vi "Data_folder_Path.vi"(1 "seconds":dbl, 2 "ProjectNumberIn":string, 3 "SetProjectNumber":bool, 4 "FlushHierarchy":bool, 5 "Data Type":string) -> (0 "Data Folder":path)   [LabVIEW 2010]
uses:
  Globals/Constants_global.vi
  Globals/Preference_global.vi
panel:
  out "ProjectNo":string
  out "Hierarchy":string[](array[string])
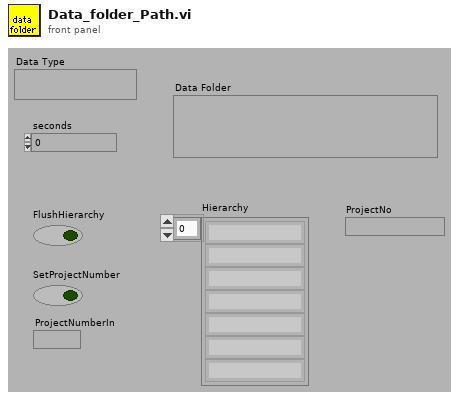
[diagram p1: front panel]
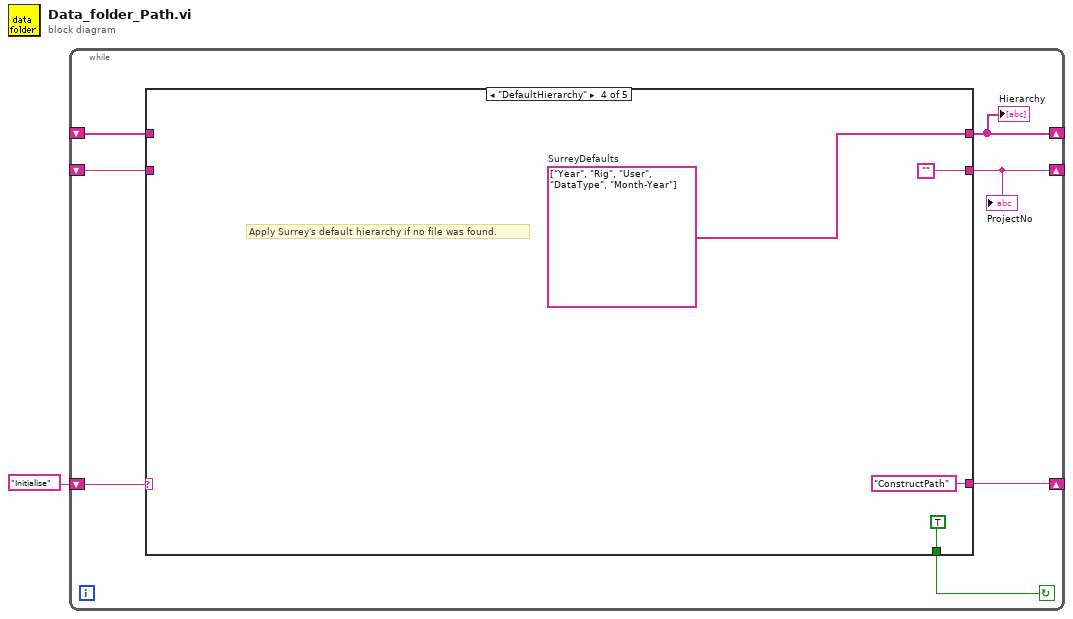
[diagram p0: block diagram]
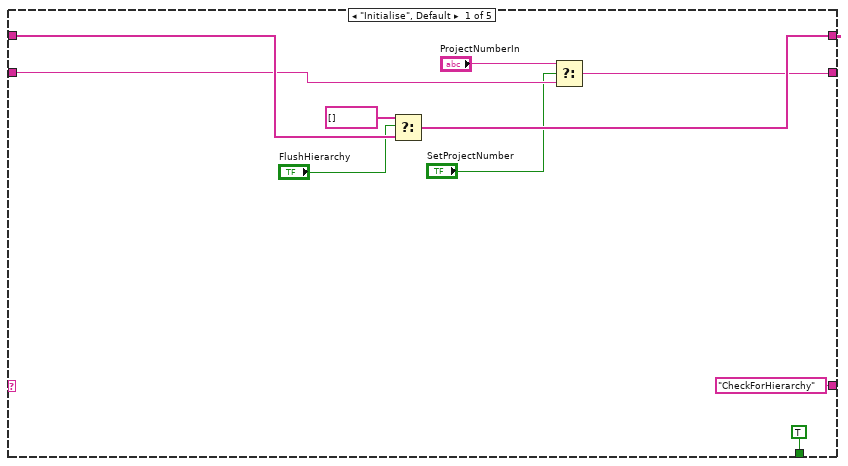
[diagram p2: hidden frame]
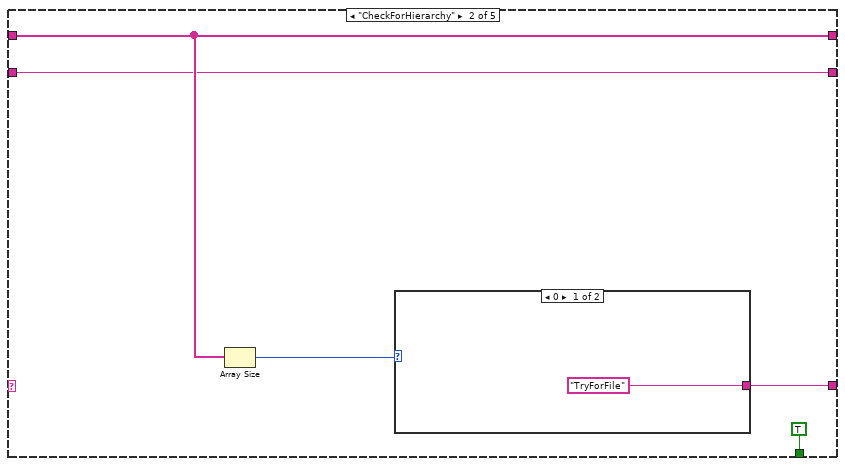
[diagram p3: hidden frame]
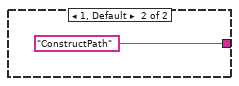
[diagram p4: hidden frame]
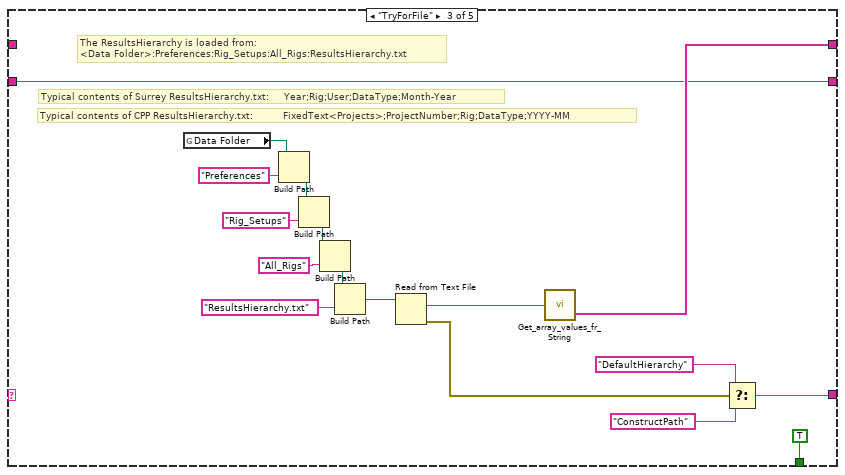
[diagram p5: hidden frame]
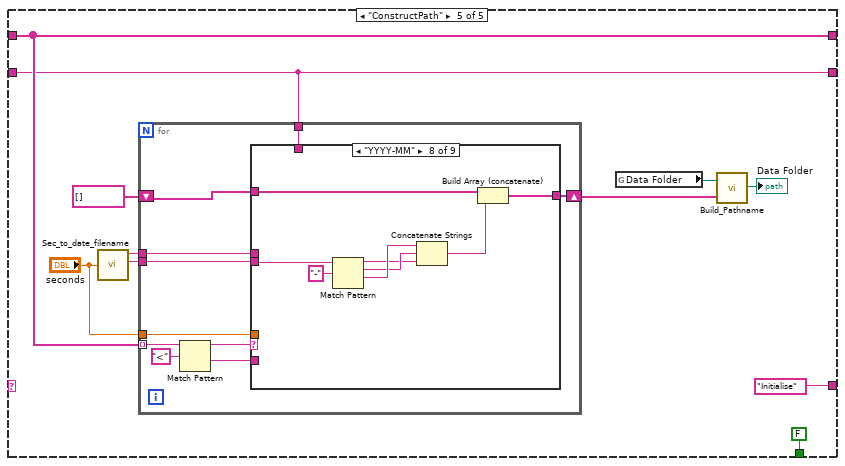
[diagram p6: hidden frame]
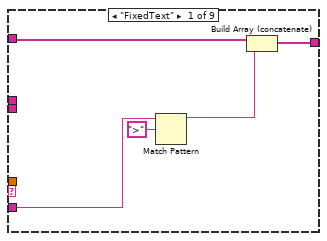
[diagram p7: hidden frame]
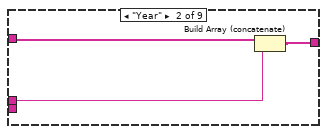
[diagram p8: hidden frame]
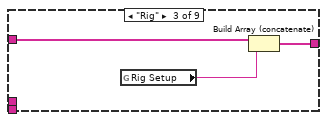
[diagram p9: hidden frame]
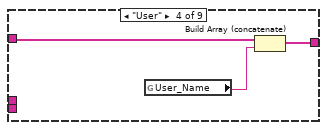
[diagram p10: hidden frame]
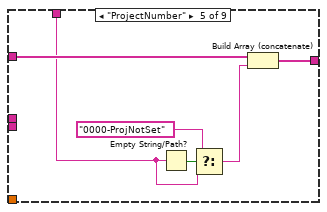
[diagram p11: hidden frame]
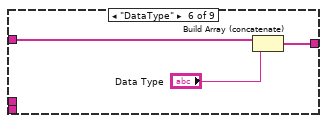
[diagram p12: hidden frame]
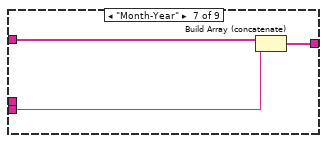
[diagram p13: hidden frame]
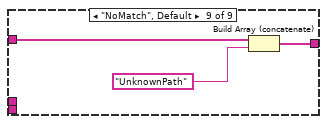
[diagram p14: hidden frame]
diagram:
  n1 = while {
    shift-right: [w6] -> _
    shift-left: _ -> [w7]
    shift-right: [w5] -> _
    shift-left: "Initialise" ("t") -> [w8]
    shift-right: [w3] -> _
    shift-left: _ -> [w4]
    stop <- w2 continue-if-true
    n2 = case shown="\"DefaultHierarchy\"" w8 {
      tunnel: w7 -> [w18 w21 _ _ w50]
      tunnel: [w17 w21 w42 w46 w50] -> w6
      tunnel: ["CheckForHierarchy" ("t") w22 w37 "ConstructPath" ("t") "Initialise" ("t")] -> w5
      tunnel: w4 -> [w12 w20 w34 _ w48]
      tunnel: [w13 w20 w34 "" ("t") w48] -> w3
      tunnel: [TRUE TRUE TRUE TRUE FALSE] -> w2
      frame "Initialise", Default {
        n3 = Select(t=string[] [], s="FlushHierarchy", f=w18) -> (s? t:f=w17:string[])
        n4 = Select(t="ProjectNumberIn", s="SetProjectNumber", f=w12) -> (s? t:f=w13:string)
      }
      frame "CheckForHierarchy" {
        n5 = Array Size(array=w21) -> (size(s)=w23:i32)
        n6 = case shown="0" w23 {
          tunnel: ["TryForFile" ("t") "ConstructPath" ("t")] -> w22
          frame 0 {
          }
          frame 1, Default {
          }
        }
      }
      frame "TryForFile" {
        # "The ResultsHierarchy is loaded from:\n<Data Folder>:Preferences:Rig_Setups:All_Rigs:ResultsHierarchy.txt"
        # "Typical contents of CPP ResultsHierarchy.txt:          FixedText<Projects>;ProjectNumber;Rig;DataType;YYYY-MM"
        # "Typical contents of Surrey ResultsHierarchy.txt:     Year;Rig;User;DataType;Month-Year"
        n7 = global read "Constants_global.vi" "Data Folder"() -> (w32:path)
        n8 = Build Path(base path=w32, name or relative path="Preferences") -> (appended path=w28:path)
        n9 = Build Path(base path=w28, name or relative path="Rig_Setups") -> (appended path=w27:path)
        n10 = Build Path(base path=w27, name or relative path="All_Rigs") -> (appended path=w39:path)
        n11 = Build Path(base path=w39, name or relative path="ResultsHierarchy.txt") -> (appended path=w31:path)
        n12 = Read from Text File(file (use dialog)=w31) -> (text=w30:string, error out=w29:errorcluster)  [unwired: 3 in, 2 out]
        n13 = call "Get_array_values_fr_String.vi"("String Value"=w30) -> ("String array"=w42:string[])  [unwired: 1 out]
        n14 = Select(t="DefaultHierarchy", s=w29, f="ConstructPath" ("t")) -> (s? t:f=w37:string)
      }
      frame "DefaultHierarchy" {
        w46 = string[] ["Year", "Rig", "User", "DataType", "Month-Year"]  # SurreyDefaults
        # "Apply Surrey's default hierarchy if no file was found."
      }
      frame "ConstructPath" {
        n15 = call "Sec_to_date_filename.vi"("seconds"="seconds") -> ("Year"=w55:string, "Month"=w54:string)  [unwired: 2 out]
        n16 = for {
          shift-right: [w67] -> w53
          shift-left: string[] [] -> [w66]
          tunnel: w50 -> [w62] mode=indexing
          tunnel: w54 -> [w65]
          tunnel: w55 -> [w64]
          tunnel: "seconds" -> [w63]
          tunnel: w48 -> [w58]
          n17 = Match Pattern(string=w62, regular expression="<") -> (before substring=w61:string, after substring=w59:string)  [unwired: 1 in, 2 out]
          n18 = case shown="\"YYYY-MM\"" w61 {
            tunnel: [w72 w75 w77 w81 w87 w90 w93 w99 w104] -> w67
            tunnel: w66 -> [w71 w74 w76 w79 w86 w89 w92 w98 w103]
            tunnel: w65 -> [_ _ _ _ _ _ w91 w101 _]
            tunnel: w64 -> [_ w73 _ _ _ _ _ _ _]
            tunnel: w63 -> [_ _ _ _ _ _ _ _ _]
            tunnel: w59 -> [w70 _ _ _ _ _ _ _ _]
            tunnel: w58 -> [_ _ _ _ w82 _ _ _ _]
            frame "FixedText" {
              n19 = Match Pattern(string=w70, regular expression=">") -> (before substring=w68:string)  [unwired: 1 in, 3 out]
              n20 = Build Array (concatenate)(w71, w68) -> (w72:string[])
            }
            frame "Year" {
              n21 = Build Array (concatenate)(w74, w73) -> (w75:string[])
            }
            frame "Rig" {
              n22 = global read "Preference_global.vi" "Rig Setup"() -> (w78:string)
              n23 = Build Array (concatenate)(w76, w78) -> (w77:string[])
            }
            frame "User" {
              n24 = global read "Preference_global.vi" "User_Name"() -> (w80:string)
              n25 = Build Array (concatenate)(w79, w80) -> (w81:string[])
            }
            frame "ProjectNumber" {
              n26 = Empty String/Path?(string/path=w82) -> (empty?=w85:bool)
              n27 = Select(t="0000-ProjNotSet", s=w85, f=w82) -> (s? t:f=w84:string)
              n28 = Build Array (concatenate)(w86, w84) -> (w87:string[])
            }
            frame "DataType" {
              n29 = Build Array (concatenate)(w89, "Data Type") -> (w90:string[])
            }
            frame "Month-Year" {
              n30 = Build Array (concatenate)(w92, w91) -> (w93:string[])
            }
            frame "YYYY-MM" {
              n31 = Match Pattern(string=w101, regular expression="-") -> (before substring=w95:string, match substring=w96:string, after substring=w97:string)  [unwired: 1 in, 1 out]
              n32 = Concatenate Strings(w97, w96, w95) -> (w94:string)
              n33 = Build Array (concatenate)(w98, w94) -> (w99:string[])
            }
            frame "NoMatch", Default {
              n34 = Build Array (concatenate)(w103, "UnknownPath" ("element")) -> (w104:string[])
            }
          }
        }
        n35 = global read "Constants_global.vi" "Data Folder"() -> (w51:path)
        n36 = call "Build_Pathname.vi"("Output Array"=w53, "Pathname"=w51) -> ("Appended path"=→"Data Folder":path)
      }
    }
    "Hierarchy" <- w6
    "ProjectNo" <- w3
  }
